vi "SCCT Close.vi"(8 "error in (no error)":errorcluster, 11 "Publisher In":refnum<class "Publisher.lvclass">) -> (0 "error out":errorcluster)   [LabVIEW 2011]
uses:
  <vilib>/TOOLS FOR SMART MINDS/SCCT/Publisher/Publisher.lvclass
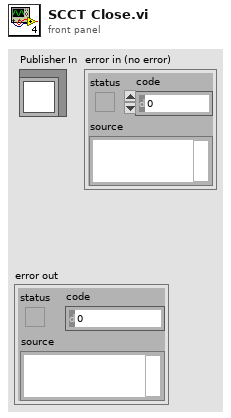
[diagram p1: front panel]
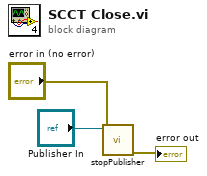
[diagram p0: block diagram]
diagram:
  n1 = call-dynamic "stopPublisher.vi"("error in (no error)"="error in (no error)", "Publisher In"="Publisher In") -> ("error out"=→"error out":errorcluster)  [unwired: 8 in, 1 out]
